vi "SendUITimeout.vi"(8 "error in (no error)":errorcluster, 11 "Queue in":refnum<queue>) -> ()   [LabVIEW 2021, in "UITimeout.lvclass"]
uses:
  UITimeout.lvclass
  AbstractionMessage/AbstractionMessage.lvclass
  C:/Users/chrismadlax/Desktop/LVSampleCode/ActorModel/AbstractionMessage/AbstractionMessage.lvclass
  UITimeout.lvclass/UITimeout.ctl
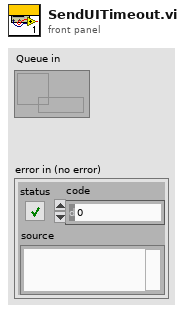
[diagram p1: front panel]
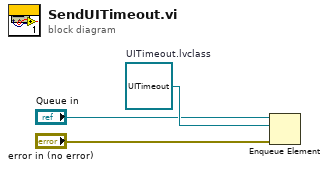
[diagram p0: block diagram]
diagram:
  w3 = refnum<class "UITimeout.lvclass"> refnum  # UITimeout.lvclass
  n1 = Enqueue Element(queue="Queue in", element=w3, error in (no error)="error in (no error)") -> ()  [unwired: 1 in, 3 out]
